vi "Real Matrix Square Root.vi"(3 "Input Matrix":T2) -> (0 "error":i32, 1 "Matrix Square Root":T1)   [LabVIEW 2020, in "NI_AALBase.lvlib"]
doc: "Computes the square root of <B>Input Matrix</B>. Wire data to the <B>Input Matrix</B> input to determine the polymorphic instance to use or manually select the instance."
uses:
  NI_AALBase.lvlib
  RealMatrix.ctl
  ComplexMatrix.ctl
  <resource>/lvanlys.dll
  NI_Matrix.lvlib
panel:
  # "Real Matrix Square Root"
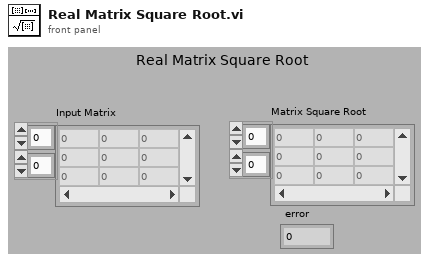
[diagram p1: front panel]
types:
  T1 = typedef "NI_Matrix.lvlib/ComplexMatrix.ctl" = cdb[][]
  T2 = typedef "NI_Matrix.lvlib/RealMatrix.ctl" = dbl[][]
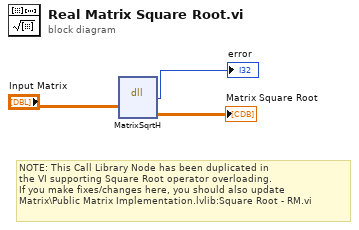
[diagram p0: block diagram]
diagram:
  # "NOTE: This Call Library Node has been duplicated in\nthe VI supporting Square Root operator overloading.\nIf you make fixes/changes here, you should also update\nMatrix\\Public Matrix Implementation.lvlib:Square Root - RM.vi"
  n1 = dll-call lib="C:/Program Files (x86)/National Instruments/LabVIEW 2020/resource/lvanlys.*" fn="MatrixSqrtH"("Input Matrix"="Input Matrix") -> (→"error":i32, "Matrix Square Root"=→"Matrix Square Root":T1)  [unwired: 5 in, 2 out]
